vi "Fit Cernox.vi"() -> ()   [LabVIEW 2018]
uses:
  <vilib>/Analysis/polynomials.llb/1D Polynomial Evaluation (DBL).vi
  <vilib>/Analysis/NI_AALPro.lvlib
panel:
  in  "R column":i32=1
  in  "T column":i32
  out "Fit coef":dbl[](array[numeric]) format="%+#_18g"
  out "Linear Graph":cluster{dbl[], dbl[]}[](graph)
  in  "Polynomial order":i32=7
  out "Log Graph":cluster{dbl[], dbl[]}[](graph)
  out "Input data":dbl[][](array[numeric])
  in  "File Path Control 2":path
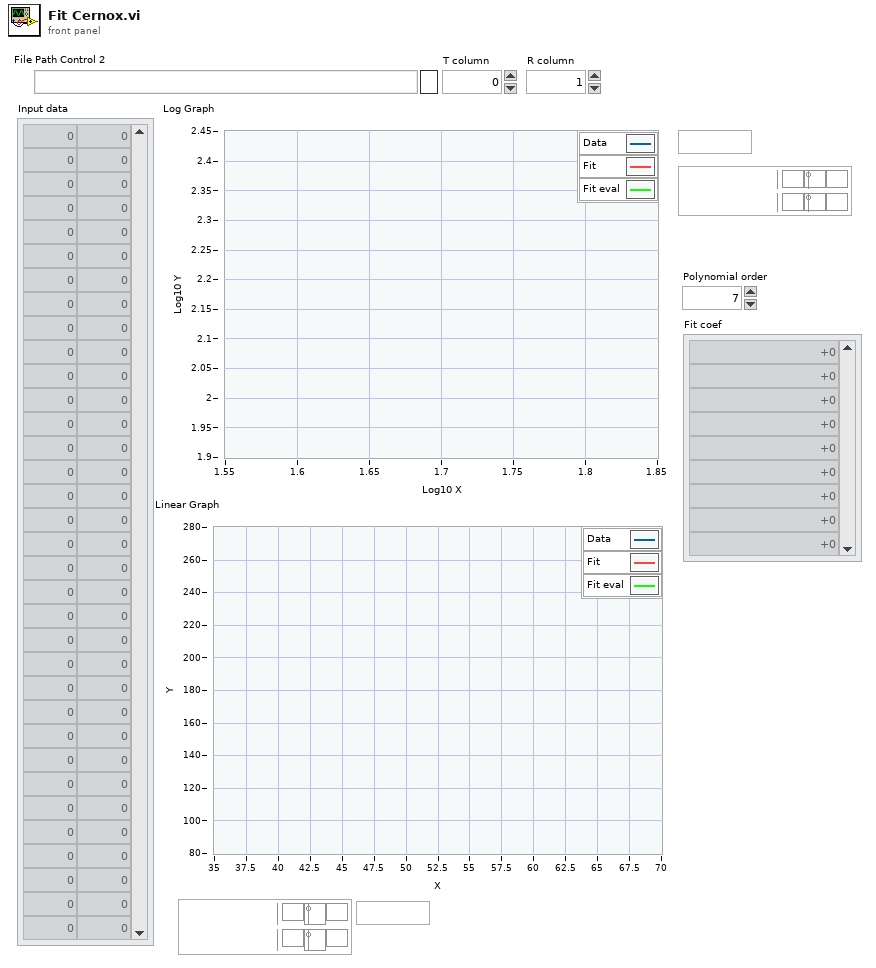
[diagram p1: front panel]
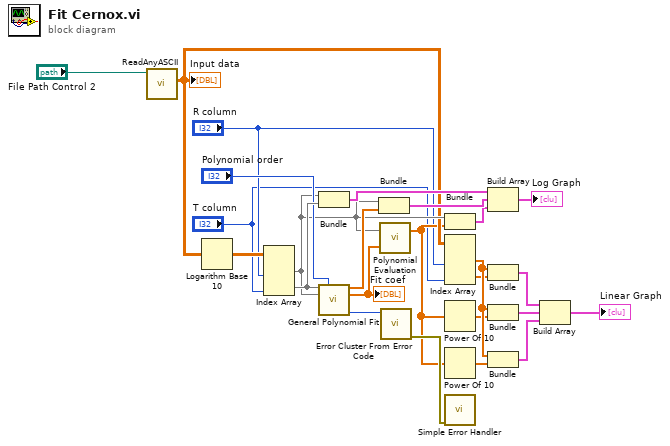
[diagram p0: block diagram]
diagram:
  n1 = call "ReadAnyASCII.vi"("file path (dialog if empty)"="File Path Control 2") -> ("all rows"=w10:dbl[][])  [unwired: 8 in, 2 out]
  "Input data" <- w10
  n2 = Logarithm Base 10(1:w10) -> (0:w23:dbl[][])
  n3 = Index Array(array=w23, index (col) #1="R column", index (col) #2="T column") -> (element #1=w14:dbl[], element #2=w22:dbl[])  [unwired: 2 in]
  n4 = Bundle(w14, w22) -> (w24:cluster{dbl[], dbl[]})  [unwired: 1 in]
  n5 = call <vilib>:"General Polynomial Fit.vi"("Y"=w22, "polynomial order"="Polynomial order", "X"=w14) -> ("Best Polynomial Fit"=w20:dbl[], "Polynomial Coefficients"=w3:dbl[], "error"=w17:i32)  [unwired: 9 in, 1 out]
  "Fit coef" <- w3
  n6 = Bundle(w14, "Best Polynomial Fit"=w20) -> (w18:cluster{dbl[], "Best Polynomial Fit":dbl[]})  [unwired: 1 in]
  n7 = call-poly <vilib>:"Polynomial Evaluation.vi"("P(x)"=w3, "A"=w14) -> ("P(A)"=w4:dbl[])  [unwired: 1 out]
  n8 = call <vilib>:"Error Cluster From Error Code.vi"("error code (0)"=w17) -> ("error out"=w16:errorcluster)  [unwired: 8 in]
  n9 = Bundle(w14, "P(A)"=w4) -> (w15:cluster{dbl[], "P(A)":dbl[]})  [unwired: 1 in]
  n10 = Index Array(array=w10, index (col) #1="R column", index (col) #2="T column") -> (element #1=w9:dbl[], element #2=w7:dbl[])  [unwired: 2 in]
  n11 = Power Of 10(x=w4) -> (10^x=w8:dbl[])
  n12 = Power Of 10(x=w4) -> (10^x=w6:dbl[])
  n13 = call <vilib>:"Simple Error Handler.vi"("error in (no error)"=w16) -> ()  [unwired: 4 in, 5 out]
  n14 = Build Array(w24, w18, w15) -> (→"Log Graph":cluster{dbl[], "P(A)":dbl[]}[])
  n15 = Bundle("all rows"=w9, "all rows"=w7) -> (w11:cluster{"all rows":dbl[], "all rows":dbl[]})  [unwired: 1 in]
  n16 = Bundle("all rows"=w9, w8) -> (w12:cluster{"all rows":dbl[], dbl[]})  [unwired: 1 in]
  n17 = Bundle("all rows"=w9, w6) -> (w13:cluster{"all rows":dbl[], dbl[]})  [unwired: 1 in]
  n18 = Build Array(w11, w12, w13) -> (→"Linear Graph":cluster{"all rows":dbl[], "all rows":dbl[]}[])
